vi "IIR Filter.vi"(10 "Filter Power":dbl, 11 "Value":dbl) -> (3 "Filtered Value":dbl)   [LabVIEW 2015]
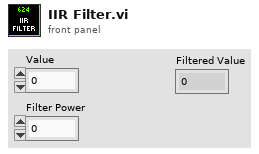
[diagram p1: front panel]
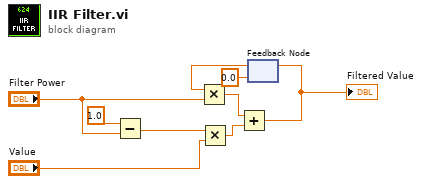
[diagram p0: block diagram]
diagram:
  n1 = Subtract(x=1.0, y="Filter Power") -> (x-y=w4:dbl)
  n2 = Multiply(x=w4, y="Value") -> (x*y=w3:dbl)
  n3 = feedback #1(0.0) -> (w7:dbl)
  n4 = Multiply(x=w7, y="Filter Power") -> (x*y=w6:dbl)
  n5 = Add(x=w6, y=w3) -> (x+y=w5:dbl)
  "Filtered Value" <- w5
  n6 = feedback-in #1(w5) -> ()
